vi "AlliGator Phasor Plot Image ROI Storage [SGL] v3.vi"(7 "Current Phasor Plot ROI Color":u32(colorbox), 8 "Error In":errorcluster, 9 "Current ROI Descriptor":T2 {"Contours"."Type" items=["No Selection", "Point", "Line", "Rectangle", "Oval", "Polygon", "Freehand Region", "Annulus", "Unused2", "Unused3", "Broken Line", "Freehand Line", "Rotated Rectangle"]}, 10 "Default Name (\"ROI\")":string="ROI", 11 "Action":T1=enum."Update Current ROI Descriptor") -> (0 "Error Out":errorcluster, 1 "Current ROI Descriptor":T2 {"Contours"."Type" items=["No Selection", "Point", "Line", "Rectangle", "Oval", "Polygon", "Freehand Region", "Annulus", "Unused2", "Unused3", "Broken Line", "Freehand Line", "Rotated Rectangle"]}, 2 "Current ROI Name":string, 3 "Current Phasor Plot Image ROI Index":i32, 4 "Old ROI Name":string, 5 "Current Phasor Plot ROI Color":u32(colorbox))   [LabVIEW 2021, in "AlliGator ROIs.lvlib"]
doc: "Handles single Phasor Plot image ROI storage."
uses:
  AlliGator ROIs.lvlib
  AlliGator ROI Manager Actions.ctl
  Globals, Variables, Constants/AlliGator Variables List.ctl
  Image/Named ROI Description.ctl
  Variant/Variant to Data/Variant to I32.vi
  GUI/GUI.lvlib
  Image/Image.lvlib
  Globals, Variables, Constants/AlliGator Globals, Variables & Constants.lvlib
  Variant/Variant to Data/Variant to Data.lvlib
  Strings/Strings.lvlib
panel:
  # "see the AlliGator License on the block diagram (Ctrl+E or Window:Show Block Diagram)"
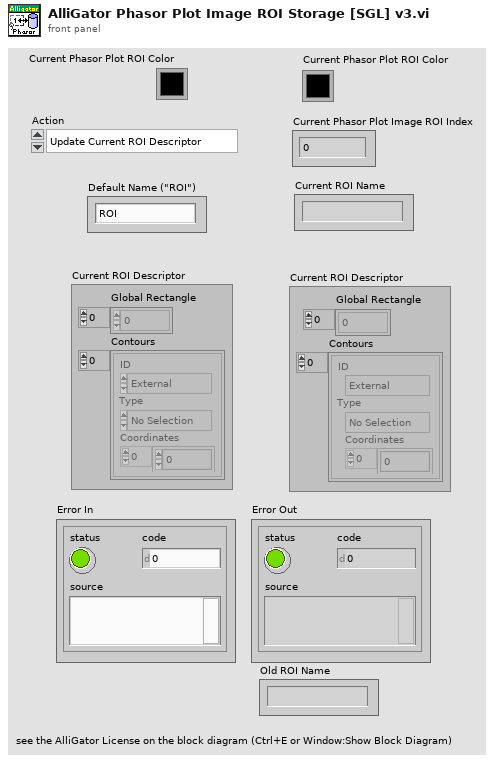
[diagram p1: front panel]
types:
  T1 = typedef "AlliGator ROIs.lvlib/AlliGator ROI Manager Actions.ctl" = enum16{"Undefined", "Delete Current ROI", "Delete All Unselected ROIs", "Delete Multiple ROIs", "Delete All ROIs", "Swap ROIs", "Insert ROI", "Update Current ROI Descriptor", "Rename Current ROI", "Store New ROI", "Store Multiple ROIs", "Select Next ROI", "Select Previous ROI", "Find Selected ROI", "Show All ROIs", "Update ROI Manager Window", "Merge All ROIs", "Unmerge ROI", "Set Selected ROI by ID"}
  T2 = typedef "ROI Descriptor" = cluster{"Global Rectangle":i32[], "Contours":cluster{"ID":enum32{"External", "Internal"}, "Type":u32, "Coordinates":i32[]}[]}
  T3 = typedef "AlliGator Globals, Variables & Constants.lvlib/AlliGator Variables List.ctl" = enum16{"---- GUI ----", "GUI:Initialization Status", "GUI:State Indicators Refnum", "GUI:Original AlliGator Menu Items", "GUI:Current Action Loop State", "GUI:Script in progress", "GUI:Playback", "GUI:Loop Playback", "GUI:Search ROI Used", "GUI:Search ROI", "Decay Graph Max Legend Size", "Intensity Graph Max Legend Size", "Decay Statistics Graph Max Legend Size", "Phasor Graph Max Legend Size", "Phasor Ratio Graph Max Legend Size", "Lifetime Graph Max Legend Size", "---- Files ----", "Files:Export Dataset Frames as Individual Files", "Files:Show Batch Export Help Balloons", "Files:Frames in Dataset", "Files:ptu File Frame Start Indices", "Files:Current Frame in Dataset", "Files:Current Frame Timestamp", "Files:Dataset Loaded", "Files:Dataset Metadata", "Files:Dataset Channel", "Files:Dataset Data Description", "Files:Background Dataset Metadata", "Files:Background Dataset Channel", "Files:Background Dataset Data Description", "Files:Background File Subtraction", "Files:Background File Path", "Files:Background File Pile-up Correction", "Files:Background File Pixel Well Capacity", "Files:Background File Scaling Factor", "Files:Current Dataset Load Settings", "Files:Dataset Path", "Files:ICCD-specific Information", "Files:Macrotime Gate Separation", "------ Python Plugins ------", "Python Plugins:Information", "Python Plugins:Python Session", "Python Plugins:Valid Python Session?", "---- Source Image ----", "Source Image:ROIs", "Source Image:Current ROI", "Source Image:ROI Event Refnum", "X_Source Image Display Range", "X_Source Image Palette Information", "X_Type of Displayed Image", "X_Time Gate Slider", "Source Image:Palette List", "Source Image:Scale", "Source Image:ROI Overlay Color", "Source Image:Overlay to Erase", "Source Image:Is Displayed Image Accumulated", "Source Image:White Light Image Modified", "Source Image:Mask Image Modified", "---- Image Profile Window ----", "Image Profile:Window Event Refnum", "Image Profile:IntensityType", "Image Profile:Intensity Average Type", "Image Profile:Intensity-weighted SDV", "Image Profile:Box Profile Type", "Image Profile:Window Open", "Image Profile:Plotted Fit Parameter", "------ Phasor Graph -------", "Phasor Graph:Show Line", "---- Phasor Plot ---", "Phasor Plot:Parameters Changed", "Phasor Plot:FLI Dataset Modified since last Calculation", "Phasor Harmonics Data", "Selected Phasor Harmonics", "Phasor Harmonic Manager Event Refnum", "Phasor Plot:ROIs", "Phasor Plot:Current ROI", "Phasor Plot:ROI Event Refnum", "Phasor Plot:Image Reference Points", "Phasor Plot:Computed", "Phasor Plot:Palette Information", "Phasor Plot:Palette List", "Phasor Plot:Phasor Ratio Palette Information", "Phasor Plot:Phasor Ratio Palette List", "Phasor Plot:Image Scale", "Phasor Plot:Image Overlay to Erase", "Phasor Plot:Image Elements to Update", "Phasor Plot:Current Calculation Parameters", "Phasor Plot:Current Calibration Options", "Phasor Plot:Reset Cumulated Phasor Plot", "Phasor Plot:Reference 1", "Phasor Plot:Lifetime Reference 1", "Phasor Plot:Reference 1 Frequency", "Phasor Plot:Reference 2", "Phasor Plot:Lifetime Reference 2", "Phasor Plot:Reference 2 Frequency", "---- Decay Analysis ----", "Number of Selected Decays to Fit", "LS Fit Results", "LAR Fit Results", "BS Fit Results", "Last Decay Max - Min", "Best Fit Parameters", "Best Fit Parameter Names", "Actual Size X", "Actual Size Y", "Binning X", "Binning Y", "Actual # Gates", "Dataset Number", "Gates to...", "Gates Skipped", "Gates to keep", "Gate Step", "Gate Separation", "Reversed Gates", "Pile-up Correction", "Pixel Well Capacity", "Background Subtracted", "Background Subtraction Method", "Background Definition Range", "Background File (deprecated)", "Number of Dataset Accumulated", "Array of Accumulated Dataset Paths", "Do Averaged Datasets", "Destination File Path", "Process Plot Target", "Use 1/D as Phasor Frequency", "---- Decay Fit Parameter Map -----", "Decay Fit Parameter Map:Palette Information", "Decay Fit Parameter Map:Palette List", "---- Parameter Map ----", "Parameter Map:Palette Information", "Parameter Map:Palette List", "------- Local Decay Window ---------", "Local Decay Graph Window:Event Refnum", "Local Decay Graph Window:Use normalized IRF for convolution", "----- Miscellaneous ----", "Misc:Skippable Dialog Windows Status"}
  T4 = typedef "Image.lvlib/Named ROI Description.ctl" = cluster{"ROI Descriptor":T2, "ROI Name":string, "Overlay Color":u32}
  T5 = typedef "AlliGator ROIs.lvlib/AlliGator Image ROI Event refnum.ctl" = refnum<user-event>
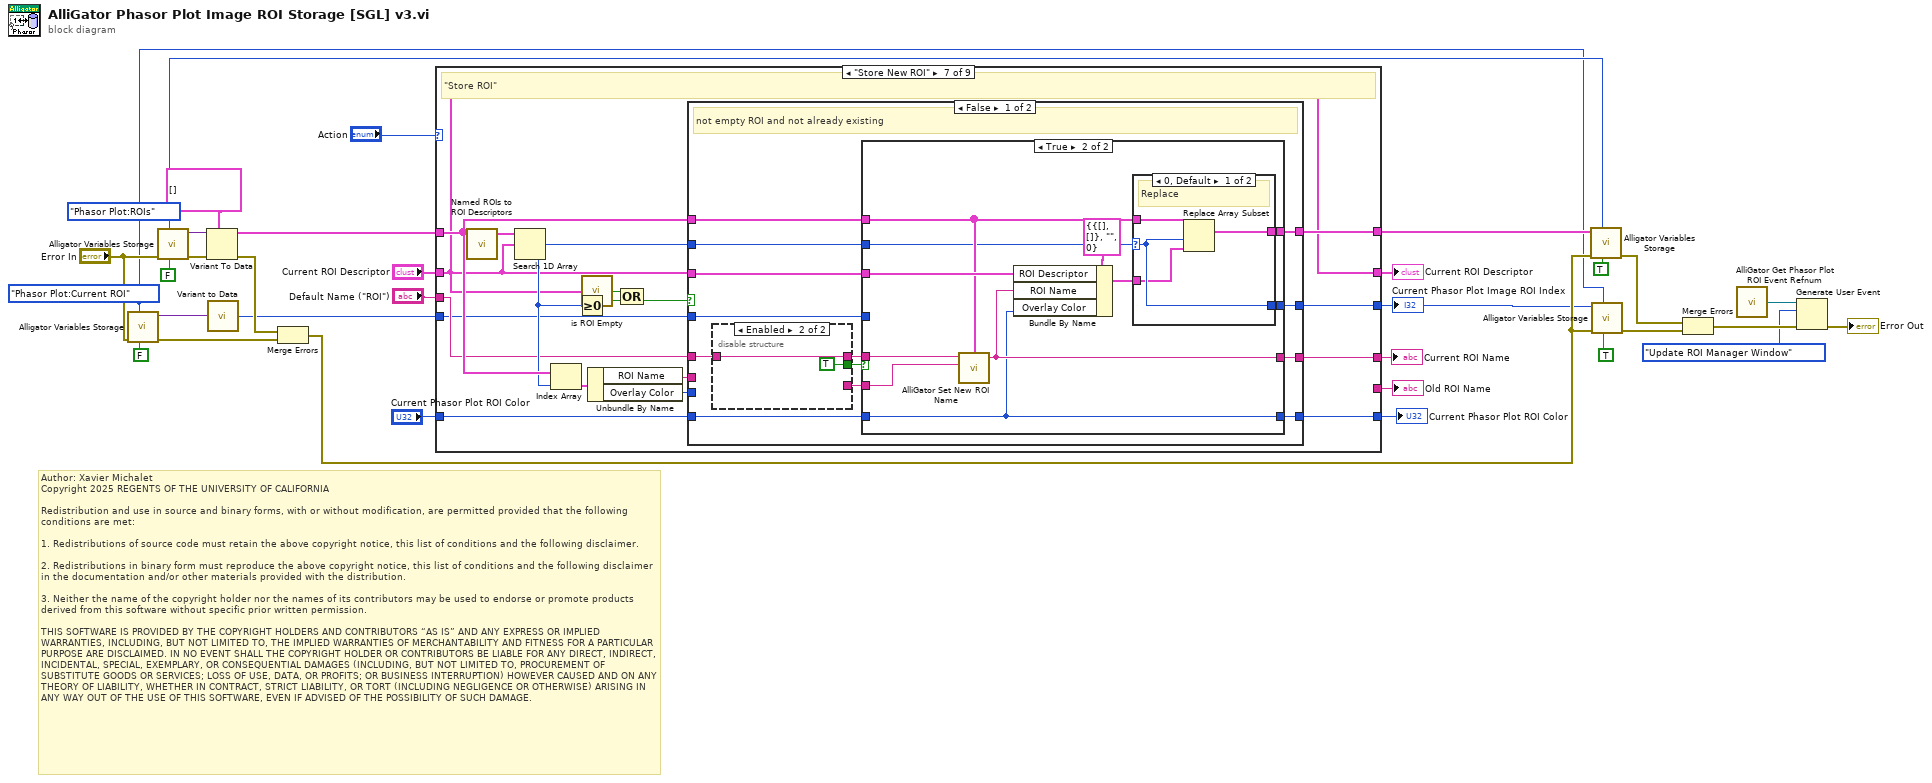
[diagram p0: block diagram]
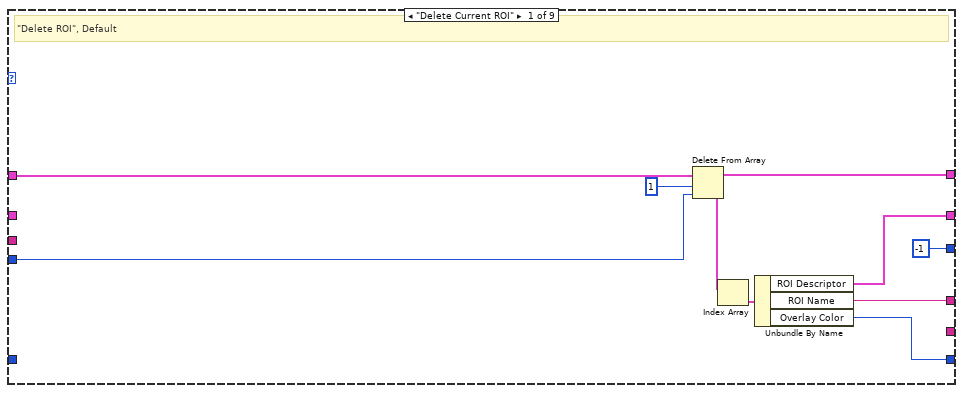
[diagram p2: hidden frame]
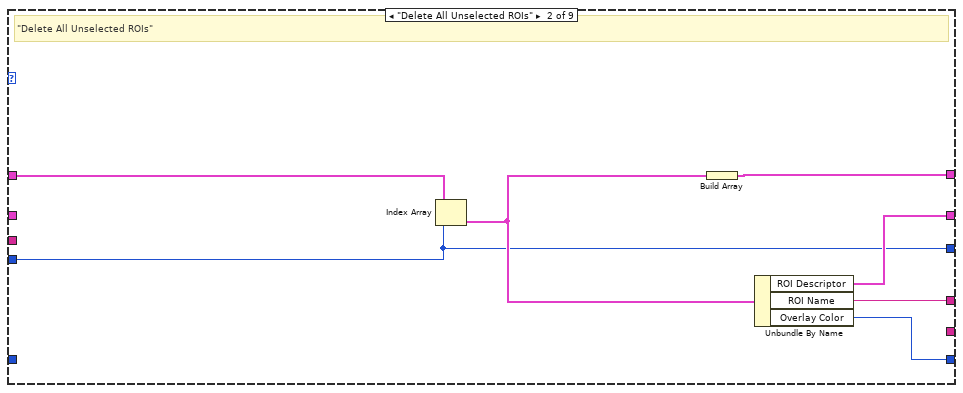
[diagram p3: hidden frame]
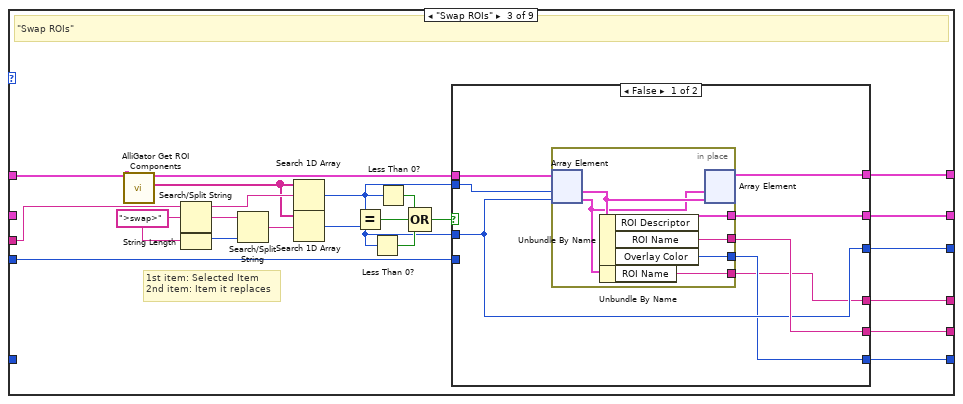
[diagram p4: hidden frame]
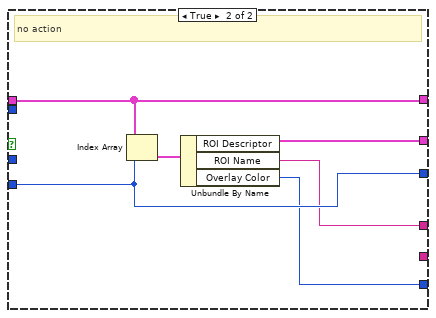
[diagram p5: hidden frame]
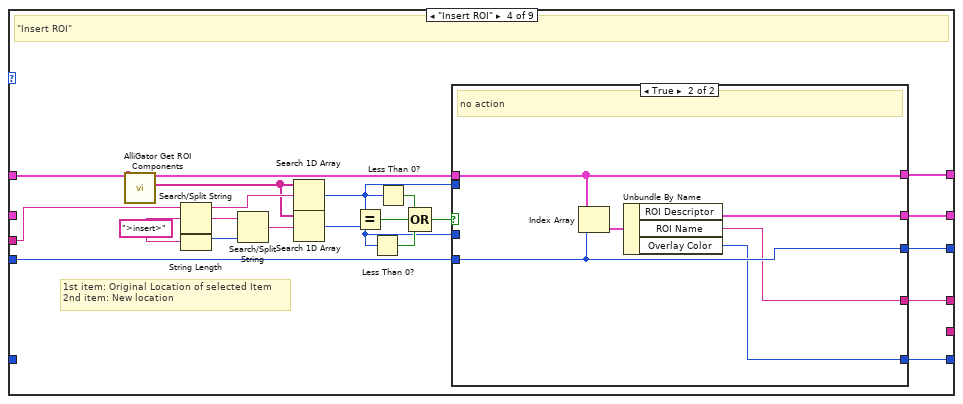
[diagram p6: hidden frame]
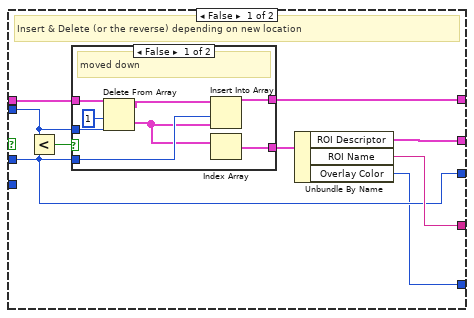
[diagram p7: hidden frame]
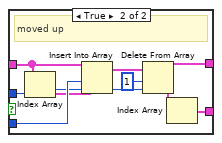
[diagram p8: hidden frame]
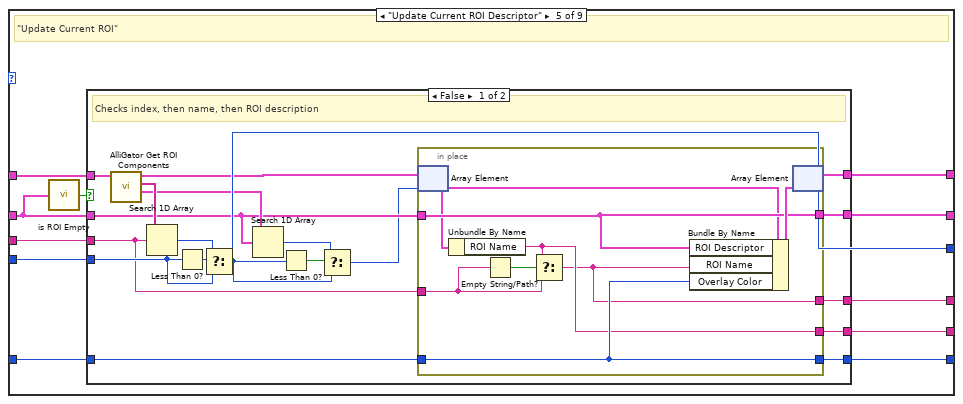
[diagram p9: hidden frame]
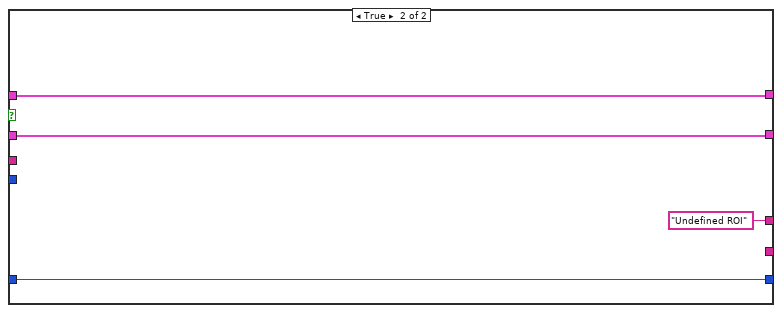
[diagram p10: hidden frame]
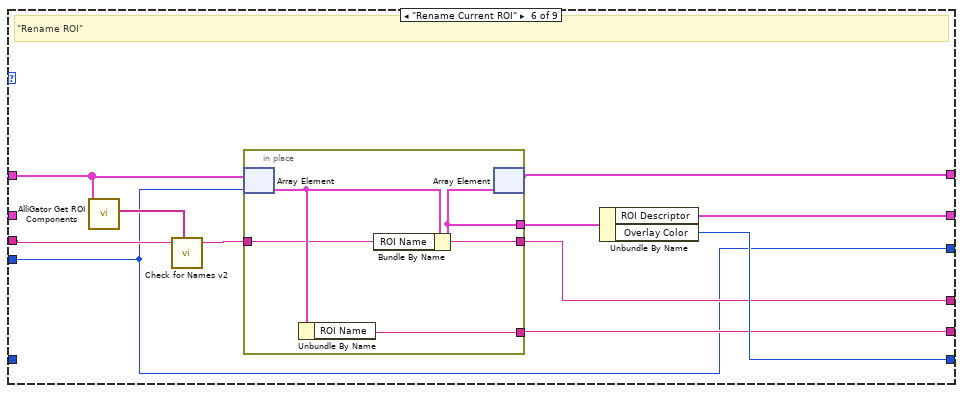
[diagram p11: hidden frame]
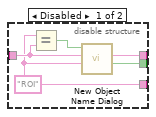
[diagram p12: hidden frame]
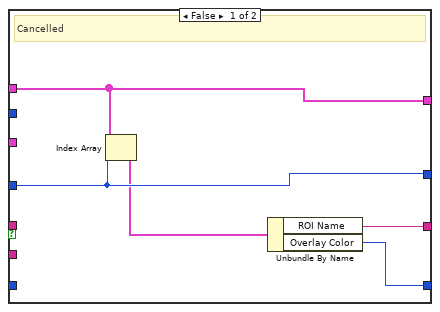
[diagram p13: hidden frame]
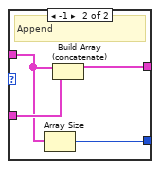
[diagram p14: hidden frame]
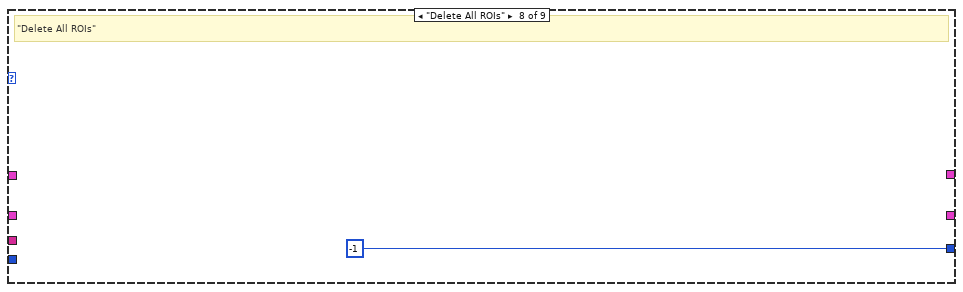
[diagram p16: hidden frame]
diagram:
  w1 = AlliGator_Variables_List."Phasor Plot:Current ROI" ("Alligator Variable")
  w2 = AlliGator_Variables_List."Phasor Plot:ROIs" ("Alligator Variable")
  # "Author: Xavier Michalet\nCopyright 2025 REGENTS OF THE UNIVERSITY OF CALIFORNIA\n\nRedistribution and use in source and binary forms, with or without modification, are permitted provided that the following conditions are met:\n\n1. Redistributions of source code must retain the above copyright notice, this list of conditions and the following disclaimer.\n\n2. Redistributions in binary form must reproduce the above copyright notice, this list of conditions and the following disclaimer in the documentation and/or other materials provided with the distribution.\n\n3. Neither the name of the copyright holder nor the names of its contributors may be used to endorse or promote products derived from this software without specific prior written permission.\n\nTHIS SOFTWARE IS PROVIDED BY THE COPYRIGHT HOLDERS AND CONTRIBUTORS “AS IS” AND ANY EXPRESS OR IMPLIED WARRANTIES, INCLUDING, BUT NOT LIMITED TO, THE IMPLIED WARRANTIES OF MERCHANTABILITY AND FITNESS FOR A PARTICULAR PURPOSE ARE DISCLAIMED. IN NO EVENT SHALL THE COPYRIGHT HOLDER OR CONTRIBUTORS BE LIABLE FOR ANY DIRECT, INDIRECT, INCIDENTAL, SPECIAL, EXEMPLARY, OR CONSEQUENTIAL DAMAGES (INCLUDING, BUT NOT LIMITED TO, PROCUREMENT OF SUBSTITUTE GOODS OR SERVICES; LOSS OF USE, DATA, OR PROFITS; OR BUSINESS INTERRUPTION) HOWEVER CAUSED AND ON ANY THEORY OF LIABILITY, WHETHER IN CONTRACT, STRICT LIABILITY, OR TORT (INCLUDING NEGLIGENCE OR OTHERWISE) ARISING IN ANY WAY OUT OF THE USE OF THIS SOFTWARE, EVEN IF ADVISED OF THE POSSIBILITY OF SUCH DAMAGE."
  n1 = call "Alligator Variables Storage.vi"("Get(F)/Set"=FALSE, "AlliGator Variable"=w1, "Error In"="Error In") -> ("Error Out"=w23:errorcluster, "Data out"=w27:variant)  [unwired: 6 in, 1 out]
  n2 = call "Alligator Variables Storage.vi"("Get(F)/Set"=FALSE, "AlliGator Variable"=w2, "Error In"="Error In") -> ("Error Out"=w31:errorcluster, "Data out"=w32:variant)  [unwired: 6 in, 1 out]
  n3 = Variant To Data(error in=w31, type=T4[] [] ("Stored ROIs in"), Variant=w32) -> (data=w16:T4[], error out=w22:errorcluster)
  n4 = call-poly "Variant to Data.vi"("Variant"=w27) -> ("Value"=w15:i32)  [unwired: 8 in]
  n5 = Merge Errors(w22, w23) -> (w17:errorcluster)
  n6 = case shown="\"Store New ROI\"" "Action" {
    tunnel: w16 -> [w42 w46 w50 w91 w153 w189 w212 _ w266]
    tunnel: w15 -> [w41 w43 w70 w110 w150 w184 w199 _ w265]
    tunnel: [w39 w45 w69 w109 w152 w188 w215 _ w266] -> w12
    tunnel: [-1 ("Current ROI out") w43 w68 w108 w150 w184 w214 -1 ("index of element") w265] -> w11
    tunnel: "Current ROI Descriptor" -> [_ _ _ _ w149 _ w206 _ w268]
    tunnel: [w34 w48 w55 w96 w151 w194 w206 _ w268] -> w10
    tunnel: "Default Name (\"ROI\")" -> [_ _ w66 w107 w143 w190 w207 _ _]
    tunnel: [w33 w47 w54 w95 w147 w186 w203 _ _] -> w9
    tunnel: [_ _ w67 _ w144 w185 _ _ _] -> w8
    tunnel: [w35 w49 w51 w92 w146 w193 w200 _ w267] -> w7
    tunnel: "Current Phasor Plot ROI Color" -> [_ _ _ _ w145 _ w201 _ w267]
    frame "Delete Current ROI" {
      # "\"Delete ROI\", Default"
      n7 = Delete From Array(array=w42, length=1, index=w41) -> (deleted portion=w37:T4[], array with subset deleted=w39:T4[])
      n8 = Index Array(array=w37) -> (element=w36:T4)  [unwired: 1 in]
      n9 = Unbundle By Name(w36) -> ("ROI Descriptor"=w34:T2, "ROI Name"=w33:string, "Overlay Color"=w35:u32)
    }
    frame "Delete All Unselected ROIs" {
      # "\"Delete All Unselected ROIs\""
      n10 = Index Array(array=w46, index=w43) -> (element=w44:T4)
      n11 = Build Array(w44) -> (w45:T4[])
      n12 = Unbundle By Name(w44) -> ("ROI Descriptor"=w48:T2, "ROI Name"=w47:string, "Overlay Color"=w49:u32)
    }
    frame "Swap ROIs" {
      w64 = ">swap>" ("search string/char (-)")
      # "1st item: Selected Item\n2nd item: Item it replaces"
      # "\"Swap ROIs\""
      n13 = call "AlliGator Get ROI Components.vi"("Stored ROIs"=w50) -> ("ROI Names"=w61:string[])  [unwired: 8 in, 2 out]
      n14 = Search/Split String(string=w66, search string/char (-)=w64) -> (substring before match=w62:string, match + rest of string=w65:string)  [unwired: 1 in, 1 out]
      n15 = String Length(string=w64) -> (length=w63:i32)
      n16 = Search/Split String(string=w65, offset (0)=w63) -> (match + rest of string=w60:string)  [unwired: 1 in, 2 out]
      n17 = Search 1D Array(1D array=w61, element=w62) -> (index of element=w53:i32)  [unwired: 1 in]
      n18 = Search 1D Array(1D array=w61, element=w60) -> (index of element=w52:i32)  [unwired: 1 in]
      n19 = Equal?(x=w53, y=w52) -> (x = y?=w57:bool)
      n20 = Less Than 0?(x=w52) -> (x < 0?=w58:bool)
      n21 = Less Than 0?(x=w53) -> (x < 0?=w59:bool)
      n22 = Compound Arithmetic op=OR(w59, w57, w58) -> (w56:bool)
      n23 = case shown="False" w56 {
        tunnel: w70 -> [_ w89]
        tunnel: [w77 w90] -> w69
        tunnel: [w73 w89] -> w68
        tunnel: [w74 _] -> w67
        tunnel: w50 -> [w78 w90]
        tunnel: [w75 w87] -> w55
        tunnel: [w71 w86] -> w54
        tunnel: w53 -> [w76 _]
        tunnel: w52 -> [w73 _]
        tunnel: [w72 w85] -> w51
        frame False {
          n24 = in-place {
            in-place-border: [w83] -> w75
            in-place-border: [w82] -> w74
            in-place-border: [w81] -> w72
            in-place-border: [w79] -> w71
            n25 = in-place-array #1(w78, w76, w73) -> (w84:T4, w80:T4)
            n26 = Unbundle By Name(w84) -> ("ROI Descriptor"=w83:T2, "ROI Name"=w82:string, "Overlay Color"=w81:u32)
            n27 = Unbundle By Name(w80) -> ("ROI Name"=w79:string)
            n28 = in-place-array #1(w80, w84) -> (w77:T4[])  [unwired: 2 out]
          }
        }
        frame True {
          # "no action"
          n29 = Index Array(array=w90, index=w89) -> (element=w88:T4)
          n30 = Unbundle By Name(w88) -> ("ROI Descriptor"=w87:T2, "ROI Name"=w86:string, "Overlay Color"=w85:u32)
        }
      }
    }
    frame "Insert ROI" {
      w105 = ">insert>" ("search string/char (-)")
      # "1st item: Original Location of selected Item\n2nd item: New location"
      # "\"Insert ROI\""
      n31 = call "AlliGator Get ROI Components.vi"("Stored ROIs"=w91) -> ("ROI Names"=w102:string[])  [unwired: 8 in, 2 out]
      n32 = Search/Split String(string=w107, search string/char (-)=w105) -> (substring before match=w103:string, match + rest of string=w106:string)  [unwired: 1 in, 1 out]
      n33 = String Length(string=w105) -> (length=w104:i32)
      n34 = Search/Split String(string=w106, offset (0)=w104) -> (match + rest of string=w101:string)  [unwired: 1 in, 2 out]
      n35 = Search 1D Array(1D array=w102, element=w103) -> (index of element=w94:i32)  [unwired: 1 in]
      n36 = Search 1D Array(1D array=w102, element=w101) -> (index of element=w93:i32)  [unwired: 1 in]
      n37 = Equal?(x=w94, y=w93) -> (x = y?=w98:bool)
      n38 = Less Than 0?(x=w93) -> (x < 0?=w99:bool)
      n39 = Less Than 0?(x=w94) -> (x < 0?=w100:bool)
      n40 = Compound Arithmetic op=OR(w100, w98, w99) -> (w97:bool)
      n41 = case shown="True" w97 {
        tunnel: w110 -> [_ w141]
        tunnel: [w116 w142] -> w109
        tunnel: [w112 w141] -> w108
        tunnel: w91 -> [w118 w142]
        tunnel: [w114 w139] -> w96
        tunnel: [w113 w138] -> w95
        tunnel: w94 -> [w117 _]
        tunnel: w93 -> [w112 _]
        tunnel: [w111 w137] -> w92
        frame False {
          # "Insert & Delete (or the reverse) depending on new location"
          n42 = Less?(x=w117, y=w112) -> (x < y?=w119:bool)
          n43 = case shown="False" w119 {
            tunnel: w118 -> [w127 w136]
            tunnel: w117 -> [w126 w132]
            tunnel: w112 -> [w122 w135]
            tunnel: [w123 w130] -> w116
            tunnel: [w120 w128] -> w115
            frame False {
              # "moved down"
              n44 = Delete From Array(array=w127, length=1, index=w126) -> (deleted portion=w121:T4[], array with subset deleted=w124:T4[])
              n45 = Insert Into Array(array=w124, index=w122, new element=w121) -> (w123:T4[])
              n46 = Index Array(array=w121) -> (element=w120:T4)  [unwired: 1 in]
            }
            frame True {
              # "moved up"
              n47 = Index Array(array=w136, index=w132) -> (element=w134:T4)
              n48 = Insert Into Array(array=w136, index=w135, new element=w134) -> (w133:T4[])
              n49 = Delete From Array(array=w133, length=1, index=w132) -> (deleted portion=w129:T4[], array with subset deleted=w130:T4[])
              n50 = Index Array(array=w129) -> (element=w128:T4)  [unwired: 1 in]
            }
          }
          n51 = Unbundle By Name(w115) -> ("ROI Descriptor"=w114:T2, "ROI Name"=w113:string, "Overlay Color"=w111:u32)
        }
        frame True {
          # "no action"
          n52 = Index Array(array=w142, index=w141) -> (element=w140:T4)
          n53 = Unbundle By Name(w140) -> ("ROI Descriptor"=w139:T2, "ROI Name"=w138:string, "Overlay Color"=w137:u32)
        }
      }
    }
    frame "Update Current ROI Descriptor" {
      # "\"Update Current ROI\""
      n54 = call "is ROI Empty.vi"("Current ROI Descriptor"=w149) -> ("Empty ROI?"=w148:bool)  [unwired: 8 in]
      n55 = case shown="False" w148 {
        tunnel: w153 -> [w164 w183]
        tunnel: [w171 w183] -> w152
        tunnel: [w170 w182] -> w151
        tunnel: [w154 "Undefined ROI" ("ROI Name")] -> w147
        tunnel: w150 -> [w165 _]
        tunnel: w149 -> [w160 w182]
        tunnel: [w167 w180] -> w146
        tunnel: w145 -> [w168 w180]
        tunnel: [w169 _] -> w144
        tunnel: w143 -> [w155 _]
        frame False {
          # "Checks index, then name, then ROI description"
          n56 = call "AlliGator Get ROI Components.vi"("Stored ROIs"=w164) -> ("ROI Descriptors"=w161:T2[], "ROI Names"=w163:string[])  [unwired: 8 in, 1 out]
          n57 = Search 1D Array(1D array=w163, element=w155) -> (index of element=w162:i32)  [unwired: 1 in]
          n58 = Less Than 0?(x=w165) -> (x < 0?=w166:bool)
          n59 = Select(t=w162, s=w166, f=w165) -> (s? t:f=w157:i32)
          n60 = Search 1D Array(1D array=w161, element=w160) -> (index of element=w158:i32)  [unwired: 1 in]
          n61 = Less Than 0?(x=w157) -> (x < 0?=w159:bool)
          n62 = Select(t=w158, s=w159, f=w157) -> (s? t:f=w156:i32)
          n63 = in-place {
            in-place-border: w160 -> [w178]
            in-place-border: [w178] -> w170
            in-place-border: [w174] -> w169
            in-place-border: w168 -> [w177]
            in-place-border: [w177] -> w167
            in-place-border: w155 -> [w173]
            in-place-border: [w172] -> w154
            n64 = in-place-array #2(w164, w156) -> (w175:T4)
            n65 = Unbundle By Name(w175) -> ("ROI Name"=w174:string)
            n66 = Empty String/Path?(string/path=w173) -> (empty?=w176:bool)
            n67 = Select(t=w174, s=w176, f=w173) -> (s? t:f=w172:string)
            n68 = Bundle By Name(cluster=w175, "ROI Descriptor"=w178, "ROI Name"=w172, "Overlay Color"=w177) -> (w179:T4)
            n69 = in-place-array #2(w179) -> (w171:T4[])  [unwired: 1 out]
          }
        }
        frame True {
        }
      }
    }
    frame "Rename Current ROI" {
      # "\"Rename ROI\""
      n70 = call "AlliGator Get ROI Components.vi"("Stored ROIs"=w189) -> ("ROI Names"=w192:string[])  [unwired: 8 in, 2 out]
      n71 = call "Check for Names v2.vi"("New Name"=w190, "Name List"=w192) -> ("New Name"=w191:string)  [unwired: 4 in, 3 out]
      n72 = in-place {
        in-place-border: w191 -> [w195]
        in-place-border: [w198] -> w187
        in-place-border: [w196] -> w185
        in-place-border: [w195] -> w186
        n73 = in-place-array #3(w189, w184) -> (w197:T4)
        n74 = Unbundle By Name(w197) -> ("ROI Name"=w196:string)
        n75 = Bundle By Name(cluster=w197, "ROI Name"=w195) -> (w198:T4)
        n76 = in-place-array #3(w198) -> (w188:T4[])  [unwired: 1 out]
      }
      n77 = Unbundle By Name(w187) -> ("ROI Descriptor"=w194:T2, "Overlay Color"=w193:u32)
    }
    frame "Store New ROI" {
      # "\"Store ROI\""
      n78 = call "Named ROIs to ROI Descriptors.vi"("Named ROIs"=w212) -> ("ROI Descriptors"=w213:T2[])  [unwired: 10 in]
      n79 = Search 1D Array(1D array=w213, element=w206) -> (index of element=w209:i32)  [unwired: 1 in]
      n80 = Index Array(array=w212, index=w209) -> (element=w211:T4)
      n81 = Greater Or Equal To 0?(x=w209) -> (x >= 0?=w208:bool)
      n82 = call "is ROI Empty.vi"("Current ROI Descriptor"=w206) -> ("Empty ROI?"=w204:bool)  [unwired: 8 in]
      n83 = Unbundle By Name(w211) -> ("ROI Name"=w210:string, "Overlay Color"=w202:u32)
      n84 = Compound Arithmetic op=OR(w204, w208) -> (w205:bool)
      n85 = case shown="False" w205 {
        tunnel: [w228 w263] -> w215
        tunnel: [w227 w261] -> w214
        tunnel: w206 -> [w226 _]
        tunnel: w212 -> [w225 w263]
        tunnel: w210 -> [_ w262]
        tunnel: w209 -> [w224 w261]
        tunnel: w207 -> [w221 _]
        tunnel: [w222 w262] -> w203
        tunnel: w202 -> [_ w260]
        tunnel: w201 -> [w216 _]
        tunnel: [w217 w260] -> w200
        tunnel: w199 -> [w218 _]
        frame False {
          # "not empty ROI and not already existing"
          n86 = disable-structure shown="Enabled" {
            disable-tunnel: [w233 w235] -> w223
            disable-tunnel: w221 -> [w231 w235]
            disable-tunnel: [w230 _] -> w220
            disable-tunnel: [w229 TRUE ("OK")] -> w219
            frame Disabled {
              w230 = "ROI" ("x")
              n87 = Equal?(x=w230, y=w231) -> (x = y?=w232:bool)
              n88 = call "New Object Name Dialog.vi"("String Name (\"object\")"=w230, "Object Name in"=w231, "Enable"=w232) -> ("OK"=w229:bool, "Object Name out"=w233:string)  [unwired: 6 in, 1 out]
            }
            frame Enabled {
            }
          }
          n89 = case shown="True" w219 {
            tunnel: [w240 w251] -> w228
            tunnel: [w239 w250] -> w227
            tunnel: w226 -> [_ w247]
            tunnel: w225 -> [w240 w246]
            tunnel: w224 -> [_ w245]
            tunnel: w223 -> [_ w244]
            tunnel: [w237 w243] -> w222
            tunnel: w220 -> [_ w242]
            tunnel: w218 -> [w239 _]
            tunnel: [w236 w241] -> w217
            tunnel: w216 -> [_ w241]
            frame False {
              # "Cancelled"
              n90 = Index Array(array=w240, index=w239) -> (element=w238:T4)
              n91 = Unbundle By Name(w238) -> ("ROI Name"=w237:string, "Overlay Color"=w236:u32)
            }
            frame True {
              n92 = call "AlliGator Set New ROI Name.vi"("Stored ROIs in"=w246, "ROI Name in"=w244, "Default Name (\"\")"=w242) -> ("ROI Name out"=w243:string)  [unwired: 6 in]
              n93 = Bundle By Name(cluster=T4 {"ROI Descriptor"={"Global Rectangle"=[], "Contours"=[]}, "ROI Name"="", "Overlay Color"=0} ("Named ROI Description"), "ROI Descriptor"=w247, "ROI Name"=w243, "Overlay Color"=w241) -> (w248:T4)
              n94 = case shown="0, Default" w245 {
                selector: w245 -> [w254 _]
                tunnel: [w253 w259] -> w251
                tunnel: [w254 w258] -> w250
                tunnel: w248 -> [w252 w257]
                tunnel: w246 -> [w255 w256]
                frame 0, Default {
                  # "Replace"
                  n95 = Replace Array Subset(array=w255, new element=w252, index=w254) -> (w253:T4[])
                }
                frame -1 {
                  # "Append"
                  n96 = Array Size(array=w256) -> (size(s)=w258:i32)
                  n97 = Build Array (concatenate)(w256, w257) -> (w259:T4[])
                }
              }
            }
          }
        }
        frame True {
          # "no need to change or empty ROI"
        }
      }
    }
    frame "Delete All ROIs" {
      # "\"Delete All ROIs\""
    }
    frame Default {
    }
  }
  "Current ROI Descriptor" <- w10
  "Current Phasor Plot Image ROI Index" <- w11
  "Current ROI Name" <- w9
  "Old ROI Name" <- w8
  "Current Phasor Plot ROI Color" <- w7
  n98 = call "Alligator Variables Storage.vi"("Get(F)/Set"=TRUE, "AlliGator Variable"=w2, "Error In"=w17, "Data in"=w12) -> ("Error Out"=w20:errorcluster)  [unwired: 5 in, 2 out]
  n99 = call "Alligator Variables Storage.vi"("Get(F)/Set"=TRUE, "AlliGator Variable"=w1, "Error In"=w17, "Data in"=w11) -> ("Error Out"=w21:errorcluster)  [unwired: 5 in, 2 out]
  n100 = Merge Errors(w20, w21) -> (w19:errorcluster)
  n101 = call "AlliGator Get Phasor Plot ROI Event Refnum.vi"() -> ("Phasor Plot ROI Event Refnum"=w4:T5)
  n102 = Generate User Event(user event=w4, event data cluster=AlliGator_ROI_Manager_Actions."Update ROI Manager Window" ("event data"), error in=w19) -> (error out=→"Error Out":errorcluster)  [unwired: 1 in, 1 out]
